vi "Get LIN Frame Type Name.vi"(11 "lin frame type id":u32) -> (3 "lin frame type name":string)   [LabVIEW 2025, in "CAN-LIN Raw Bus Capture.lvclass"]
uses:
  CAN-LIN Raw Bus Capture.lvclass
  CAN-LIN Raw Bus Capture.lvclass/CAN-LIN Raw Bus Capture.ctl
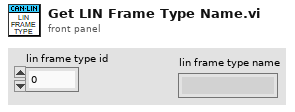
[diagram p1: front panel]
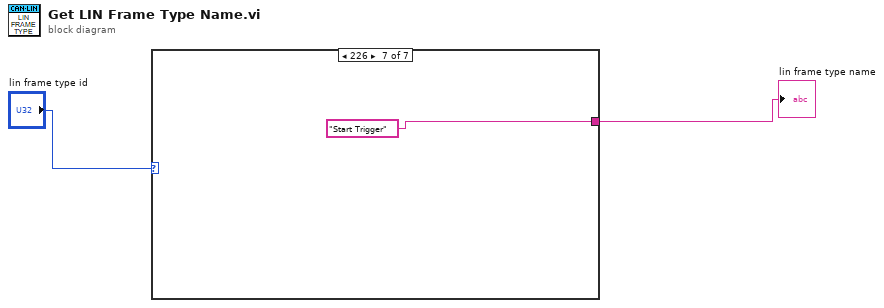
[diagram p0: block diagram]
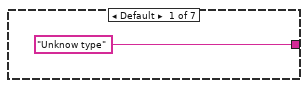
[diagram p2: hidden frame]
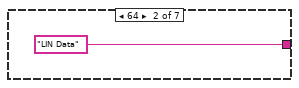
[diagram p3: hidden frame]
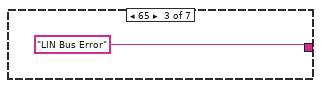
[diagram p4: hidden frame]
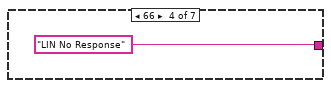
[diagram p5: hidden frame]
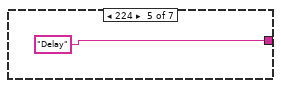
[diagram p6: hidden frame]
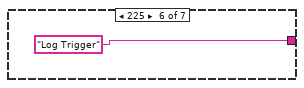
[diagram p7: hidden frame]
diagram:
  n1 = case shown="226" "lin frame type id" {
    tunnel: ["Unknow type" ("String") "LIN Data" ("String") "LIN Bus Error" ("String") "LIN No Response" ("String") "Delay" ("String") "Log Trigger" ("String") "Start Trigger" ("String")] -> w1
    frame Default {
    }
    frame 64 {
    }
    frame 65 {
    }
    frame 66 {
    }
    frame 224 {
    }
    frame 225 {
    }
    frame 226 {
    }
  }
  "lin frame type name" <- w1
